vi "Build Transfer ID.vi"(10 "SDI":u8 format="%03b", 11 "label":T1 format="%08b") -> (3 "transfer ID":u32 format="%010b")   [LabVIEW 2020]
uses:
  Label.ctl
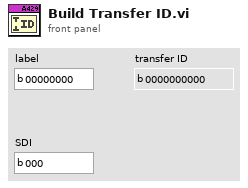
[diagram p1: front panel]
types:
  T1 = typedef "Label.ctl" = u8
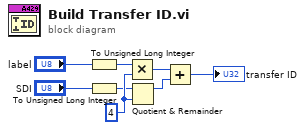
[diagram p0: block diagram]
diagram:
  w6 = u32 4 ("y")
  n1 = To Unsigned Long Integer(number="label") -> (unsigned 32bit integer=w5:u32)
  n2 = To Unsigned Long Integer(number="SDI") -> (unsigned 32bit integer=w4:u32)
  n3 = Multiply(x=w5, y=w6) -> (x*y=w2:u32)
  n4 = Quotient & Remainder(x=w4, y=w6) -> (x-y*floor(x/y)=w3:u32)  [unwired: 1 out]
  n5 = Add(x=w2, y=w3) -> (x+y=→"transfer ID":u32)
